vi "Initialize Fake Hardware Custom Device.vi"(8 "error in (no error)":errorcluster, 11 "Hardware Ref in":T1 format="%.0x") -> (0 "error out":errorcluster, 3 "Hardware Ref out":T1 format="%.0x")   [LabVIEW 2017, in "Fake Hardware Custom Device.lvlib"]
uses:
  Fake Hardware Custom Device.lvlib
  <vilib>/NI Veristand/Custom Device API/Custom Device Item Ref.ctl
  Shared/Routing and Faulting Hardware API/Types/Possible Connections for Endpoint.ctl
  Shared/Routing and Faulting Hardware API/Routing and Faulting Hardware API.lvlib
  <vilib>/NI Veristand/Custom Device API/Custom Device API.lvlib
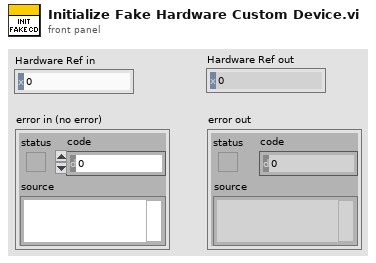
[diagram p1: front panel]
types:
  T1 = typedef "Custom Device API.lvlib/Custom Device Item Ref.ctl" = u64
  T2 = typedef "Routing and Faulting Hardware API.lvlib/Possible Connections for Endpoint.ctl" = cluster{"Source":string, "Destinations":string[]}
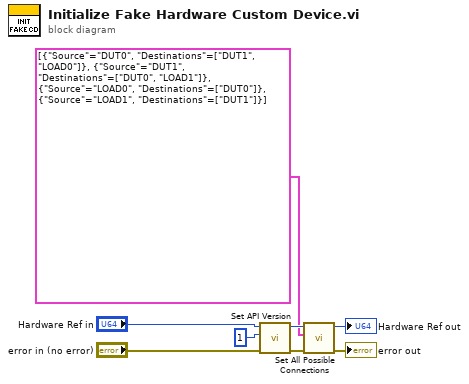
[diagram p0: block diagram]
diagram:
  n1 = call "Set API Version.vi"("error in (no error)"="error in (no error)", "API version"=u32 1, "Hardware Ref in"="Hardware Ref in") -> ("error out"=w4:errorcluster, "Hardware Ref out"=w5:T1)  [unwired: 7 in]
  n2 = call "Set All Possible Connections.vi"("error in (no error)"=w4, "Possible Connections"=T2[] [{"Source"="DUT0", "Destinations"=["DUT1", "LOAD0"]}, {"Source"="DUT1", "Destinations"=["DUT0", "LOAD1"]}, {"Source"="LOAD0", "Destinations"=["DUT0"]}, {"Source"="LOAD1", "Destinations"=["DUT1"]}], "Hardware Ref in"=w5) -> ("error out"=→"error out":errorcluster, "Hardware Ref out"=→"Hardware Ref out":T1)  [unwired: 7 in]
